vi "getColors.vi"(8 "error in (no error)":errorcluster, 11 "Theme in":refnum<class "Theme.lvclass">) -> (0 "error out":errorcluster, 2 "Colors":T1, 3 "Theme out":refnum<class "Theme.lvclass">)   [LabVIEW 2017, in "Theme.lvlib" / "Theme.lvclass"]
uses:
  Theme.lvclass
  Theme.Colors/Colors.ctl
  Theme.lvclass/Theme.ctl
  Theme.Colors/Theme.Colors.lvclass/Theme.Colors.ctl
  Theme.Colors/getContainer.vi
  Theme.Colors/getMain.vi
  Theme.Colors/getText.vi
  Theme.Colors/Theme.Colors.lvclass
  Theme.Font/Theme.Font.lvclass
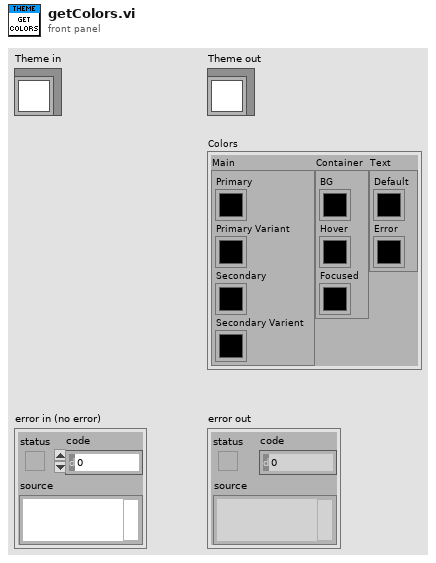
[diagram p1: front panel]
types:
  T1 = typedef "Theme.lvlib/Theme.Colors.lvclass/Colors.ctl" = cluster{"Main":cluster{"Primary":u32, "Primary Variant":u32, "Secondary":u32, "Secondary Varient":u32}, "Container":cluster{"BG":u32, "Hover":u32, "Focused":u32}, "Text":cluster{"Default":u32, "Error":u32}}
  T2 = typedef "Theme.lvlib/Theme.lvclass/Private Data.ctl" = cluster{"Colors":refnum<class "Theme.Colors.lvclass">, "Font":refnum<class "Theme.Font.lvclass">}
  T3 = cluster{"Primary":u32, "Primary Variant":u32, "Secondary":u32, "Secondary Varient":u32}
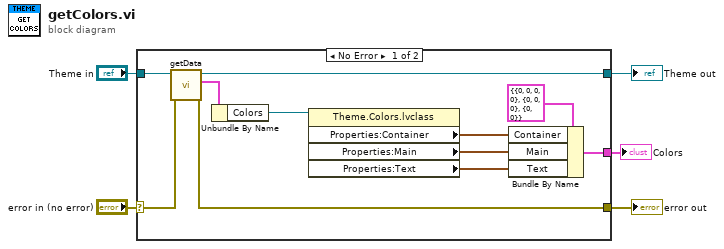
[diagram p0: block diagram]
diagram:
  n1 = case shown="No Error" "error in (no error)" {
    selector: "error in (no error)" -> [w12 w18]
    tunnel: [w11 w18] -> w4
    tunnel: [w15 w17] -> w2
    tunnel: "Theme in" -> [w16 w17]
    tunnel: [w6 _] -> w1
    frame No Error {
      n2 = call "getData.vi"("error in (no error)"=w12, "Theme in"=w16) -> ("error out"=w11:errorcluster, "Theme"=w14:T2, "Theme out"=w15:refnum<class "Theme.lvclass">)  [unwired: 7 in]
      n3 = Unbundle By Name(w14) -> ("Colors"=w13:refnum<class "Theme.Colors.lvclass">)
      n4 = property class="Theme.Colors.lvclass"(reference=w13) -> ("Properties:Container"=w7:cluster{"BG":u32, "Hover":u32, "Focused":u32}, "Properties:Main"=w8:T3, "Properties:Text"=w9:cluster{"Default":u32, "Error":u32})  [unwired: 1 in, 2 out]
      n5 = Bundle By Name(cluster=T1 {"Main"={"Primary"=0, "Primary Variant"=0, "Secondary"=0, "Secondary Varient"=0}, "Container"={"BG"=0, "Hover"=0, "Focused"=0}, "Text"={"Default"=0, "Error"=0}} ("Filled Text Fields.Theme"), "Container"=w7, "Main"=w8, "Text"=w9) -> (w6:T1)
    }
    frame Error {
    }
  }
  "error out" <- w4
  "Theme out" <- w2
  "Colors" <- w1
